vi "MDPtr SetCopyCount.vi"(8 "Copy Count":i32, 9 "error in (no error)":errorcluster, 10 "HexStrPtr":T1) -> (2 "error out":errorcluster, 3 "HexStrPtr (dup)":T1)   [LabVIEW 2014]
uses:
  MDPtr TypeDef/MDPtr.ctl
  MDPtr TypeDef/MDPtr DataFrame-PlaceHolder.ctl
  MDPtr TypeDef/MDPtr DataFrame-Common.ctl
  MDPtr TypeDef/MDPtr SupportedDataTypeDef.ctl
  <userlib>/_OpenG.lib/error/error.llb/Build Error Cluster__ogtk.vi
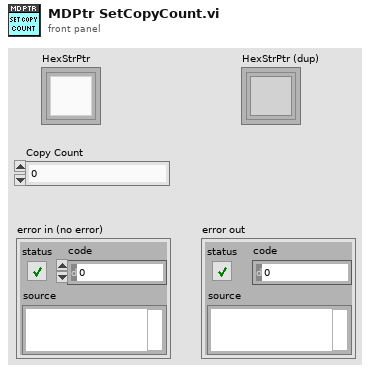
[diagram p1: front panel]
types:
  T1 = typedef "MDPtr.ctl" = refnum<k1>
  T2 = typedef "MDPtr DataFrame-PlaceHolder.ctl" = cluster{"Common":T3, "DVR":refnum<data-value>}
  T3 = typedef "MDPtr DataFrame-Common.ctl" = cluster{"Data Type":T4, "Copy Count":i32}
  T4 = typedef "MDPtr SupportedDataTypeDef.ctl" = enum16{"<Invalid>", "Waveform", "Waveform Arr", "Double Arr"}
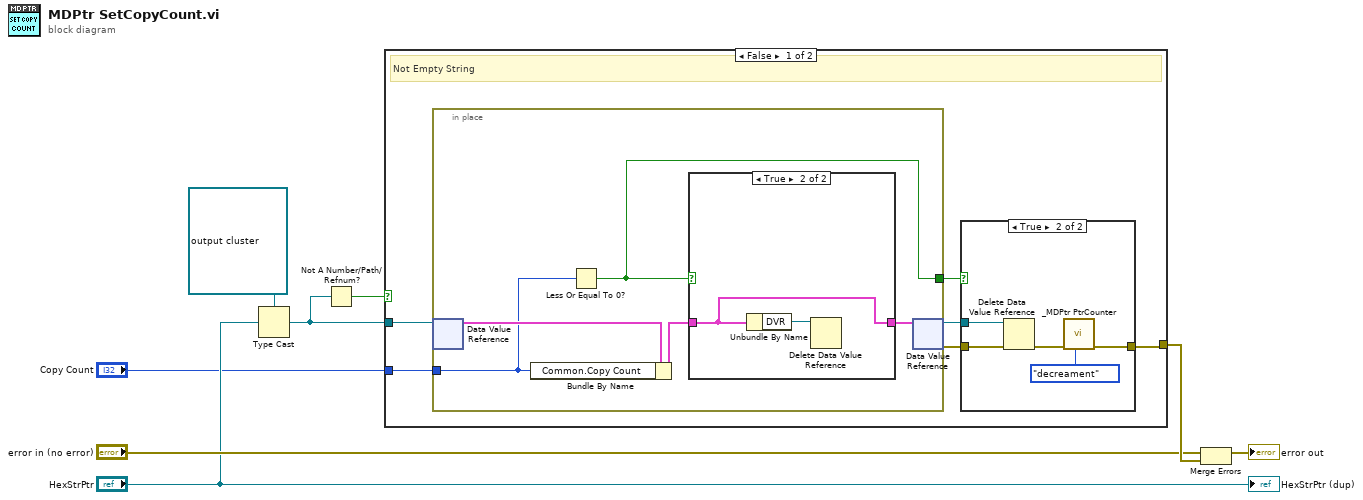
[diagram p0: block diagram]
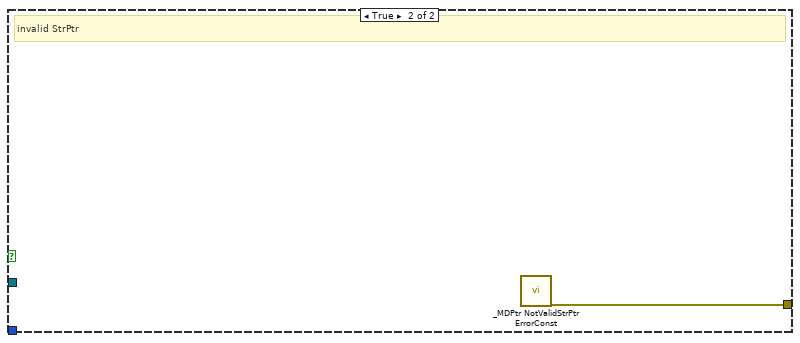
[diagram p4: hidden frame]
diagram:
  n1 = Type Cast(type=refnum<data-value> refnum ("data value reference"), x="HexStrPtr") -> (*(type *) &x=w2:refnum<data-value>)
  n2 = Not A Number/Path/Refnum?(number/path/refnum=w2) -> (NaN/Path/Refnum?=w3:bool)
  n3 = case shown="False" w3 {
    tunnel: [w11 w29] -> w8
    tunnel: w2 -> [w13 _]
    tunnel: "Copy Count" -> [w12 _]
    frame False {
      # "Not Empty String"
      n4 = in-place {
        in-place-border: w12 -> [w22]
        in-place-border: [w21] -> w9
        n5 = in-place-dvr #1(w13) -> (w25:T2)  [unwired: 1 out]
        n6 = Bundle By Name(cluster=w25, "Common.Copy Count"=w22) -> (w24:T2)
        n7 = Less Or Equal To 0?(x=w22) -> (x <= 0?=w21:bool)
        n8 = case shown="True" w21 {
          tunnel: w24 -> [w26 w27]
          tunnel: [w26 w27] -> w23
          frame False {
          }
          frame True {
            n9 = Unbundle By Name(w27) -> ("DVR"=w28:refnum<data-value>)
            n10 = Delete Data Value Reference(data value reference=w28) -> ()  [unwired: 1 in, 2 out]
          }
        }
        n11 = in-place-dvr #1(w23) -> (w10:refnum<data-value>, w14:errorcluster)
      }
      n12 = case shown="True" w9 {
        tunnel: w14 -> [w15 w20]
        tunnel: [w15 w17] -> w11
        tunnel: w10 -> [_ w18]
        frame False {
        }
        frame True {
          n13 = Delete Data Value Reference(data value reference=w18, error in=w20) -> (error out=w19:errorcluster)  [unwired: 1 out]
          n14 = call "_MDPtr PtrCounter.vi"("Oper(Get)"=enum16{"GET", "Increament", "decreament"}."decreament", "error in (no error)"=w19) -> ("error out"=w17:errorcluster)  [unwired: 8 in, 1 out]
        }
      }
    }
    frame True {
      # "invalid StrPtr"
      n15 = call "_MDPtr NotValidStrPtr ErrorConst.vi"() -> ("error out"=w29:errorcluster)  [unwired: 19 in]
    }
  }
  n16 = Merge Errors("error in (no error)", w8) -> (→"error out":errorcluster)
  "HexStrPtr (dup)" <- "HexStrPtr"
